vi "Modbus LDO Time Display.vi"(6 "Counter of oil injections 1.1 cc/min":u16, 9 "Blower ON/OFF":bool, 10 "Absolute Time":dbl, 11 "Timing in":T1 {"Absolute Time" format="%<%H:%M:%S%3u>t"; "Display Time" format="%#.20f"; "Test Time Ref" format="%#.20f"; "Precondition Time Ref" format="%#.20f"; "First Call Time Ref" format="%#.20f"}) -> (3 "Timing Out":T1 {"Absolute Time" format="%<%H:%M:%S%3u>t"; "Display Time" format="%#.20f"; "Test Time Ref" format="%#.20f"; "Precondition Time Ref" format="%#.20f"; "First Call Time Ref" format="%#.20f"})   [LabVIEW 2023, in "Modbus.lvlib"]
uses:
  Modbus.lvlib
  Modbus Timing.ctl
  <vilib>/Utility/miscctls.llb/LVDateTimeRec.ctl
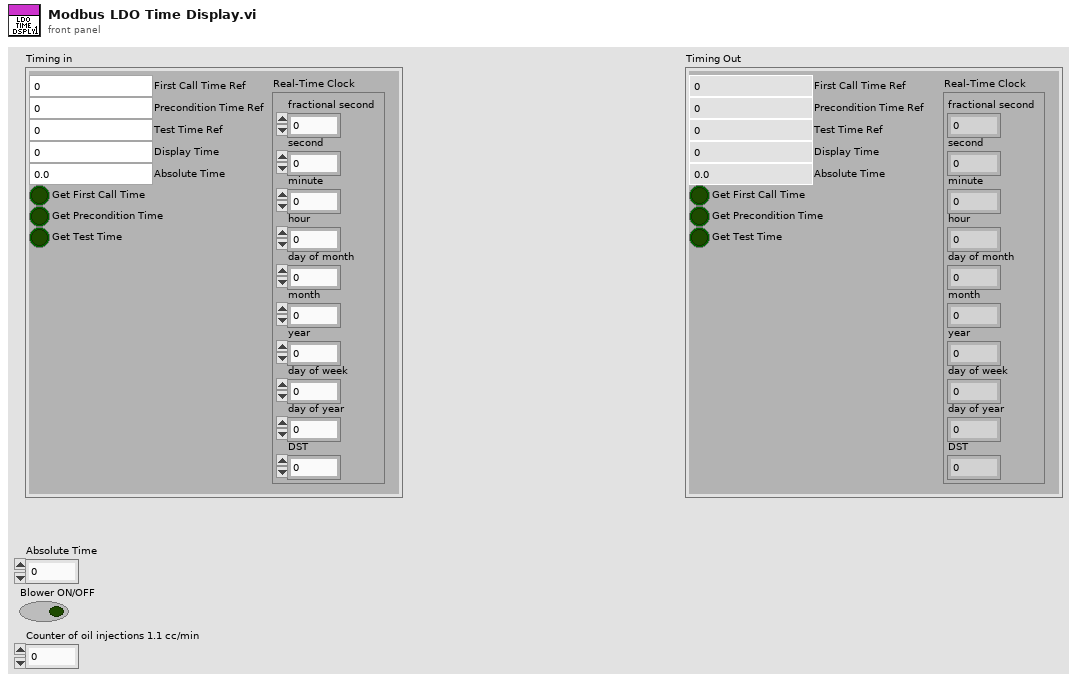
[diagram p1: front panel]
types:
  T1 = typedef "Modbus Timing.ctl" = cluster{"First Call Time Ref":dbl, "Precondition Time Ref":dbl, "Test Time Ref":dbl, "Get First Call Time":bool, "Get Precondition Time":bool, "Get Test Time":bool, "Display Time":dbl, "Real-Time Clock":T2, "Absolute Time":dbl}
  T2 = typedef "LVDateTimeRec.ctl" = cluster{"fractional second":dbl, "second":i32, "minute":i32, "hour":i32, "day of month":i32, "month":i32, "year":i32, "day of week":i32, "day of year":i32, "DST":i32}
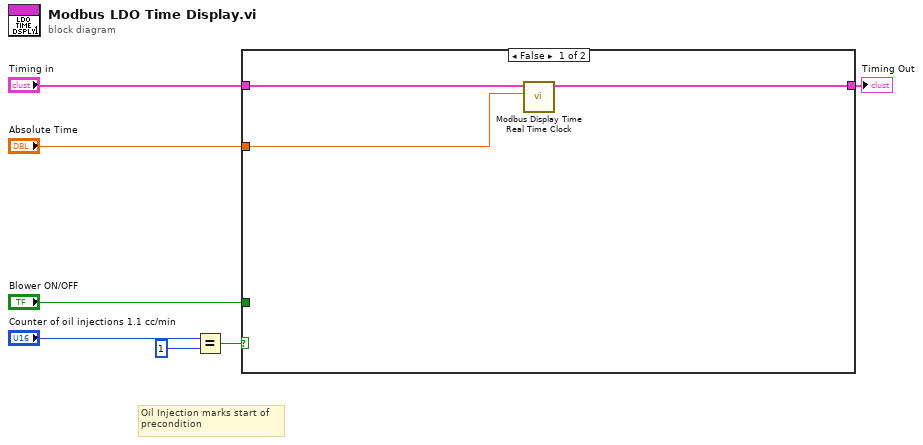
[diagram p0: block diagram]
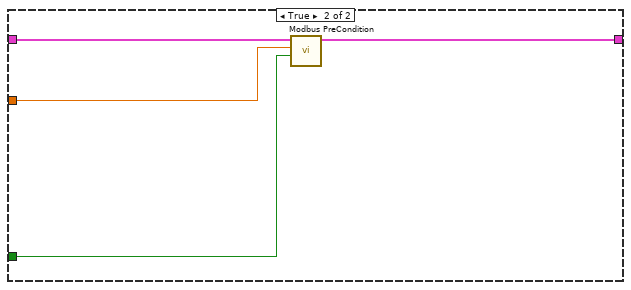
[diagram p2: hidden frame]
diagram:
  # "Oil Injection marks start of \nprecondition"
  n1 = Equal?(x="Counter of oil injections 1.1 cc/min", y=u16 1) -> (x = y?=w5:bool)
  n2 = case shown="False" w5 {
    tunnel: "Absolute Time" -> [w10 w12]
    tunnel: "Timing in" -> [w9 w14]
    tunnel: [w8 w13] -> w3
    tunnel: "Blower ON/OFF" -> [_ w11]
    frame False {
      n3 = call "Modbus Display Time Real Time Clock.vi"("Absolute Time"=w10, "Timing in in"=w9) -> ("Timing out"=w8:T1)  [unwired: 9 in]
    }
    frame True {
      n4 = call "Modbus PreCondition.vi"("Blower ON/OFF"=w11, "Absolute Time"=w12, "Timing in"=w14) -> ("Timing Out"=w13:T1)  [unwired: 8 in]
    }
  }
  "Timing Out" <- w3
